vi "Save messages PGserver.vi"(7 "stop":bool, 8 "error in":errorcluster, 9 "write enable":bool=TRUE, 10 "msg":refnum<queue>, 11 "SP in":refnum<class "Save messages PGserver.lvclass">) -> (0 "error out":errorcluster, 2 "stopped":bool, 3 "SP out":refnum<class "Save messages PGserver.lvclass">)   [LabVIEW 2019, in "Save messages PGserver.lvclass"]
uses:
  Save messages PGserver.lvclass
  ctl/Save_prog_State.ctl
  Save messages PGserver.lvclass/Save messages PGserver.ctl
  PostgreSQL2LabVIEW/libpqUtility64/src/PQclose.vi
  Modbus/Eth Status/Eth Status Read Error.vi
  PostgreSQL2LabVIEW/libpqUtility64/src/PQexecute.vi
  Read conn.vi
  PostgreSQL2LabVIEW/libpqlv64/src/PQfinish.vi
  PostgreSQL2LabVIEW/libpqlv64/src/PQresultErrorMessage.vi
  PostgreSQL2LabVIEW/libpqUtility64/src/PQclear.vi
  PostgreSQL2LabVIEW/libpqlv64/src/PQsendQuery.vi
  PostgreSQL2LabVIEW/libpqlv64/src/PQgetResult.vi
  PostgreSQL2LabVIEW/libpqlv64/src/PQresultStatus.vi
  PostgreSQL2LabVIEW/libpqlv64/src/PQclear.vi
  Timer Delay/Timers.lvlib
  Modbus/Eth Status/Eth Status.lvlib
  PostgreSQL.lvlib
panel:
  out "t ms":u32
  out "State":T1=enum."requests"
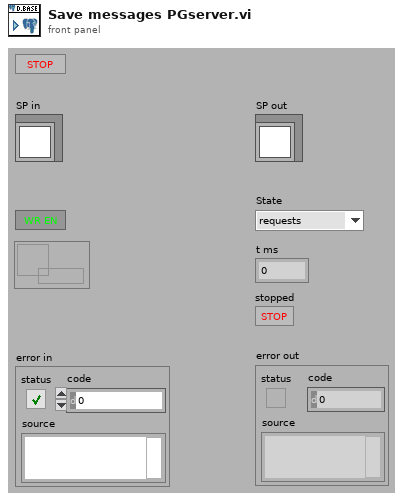
[diagram p1: front panel]
types:
  T1 = typedef "PostgreSQL.lvlib/Save_prog_State.ctl" = enum8{"initialization", "redefine", "standby", "connect", "wait to reconnect", "wait to reset timeout", "configure", "requests", "close connection", "stop"}
  T2 = typedef "Eth Status.lvlib/ICPCON Status.ctl" = cluster{"Set_state_com":refnum<data-value>, "start":refnum<data-value>, "WrEn":refnum<data-value>, "errors":refnum<data-value>, "connect":refnum<data-value>, "state":refnum<data-value>}
  T3 = typedef "PostgreSQL.lvlib/Coninfo.ctl" = cluster{"host":string, "port":string, "client_encoding":string, "dbname":string, "user":string, "password":string}
  T4 = typedef "PostgreSQL.lvlib/Save_prog_timeouts.ctl" = cluster{"reconn_timeout":i32, "read_timeout":i32, "N attempt max":i32, "t_reset_TTL":i32, "period":i32}
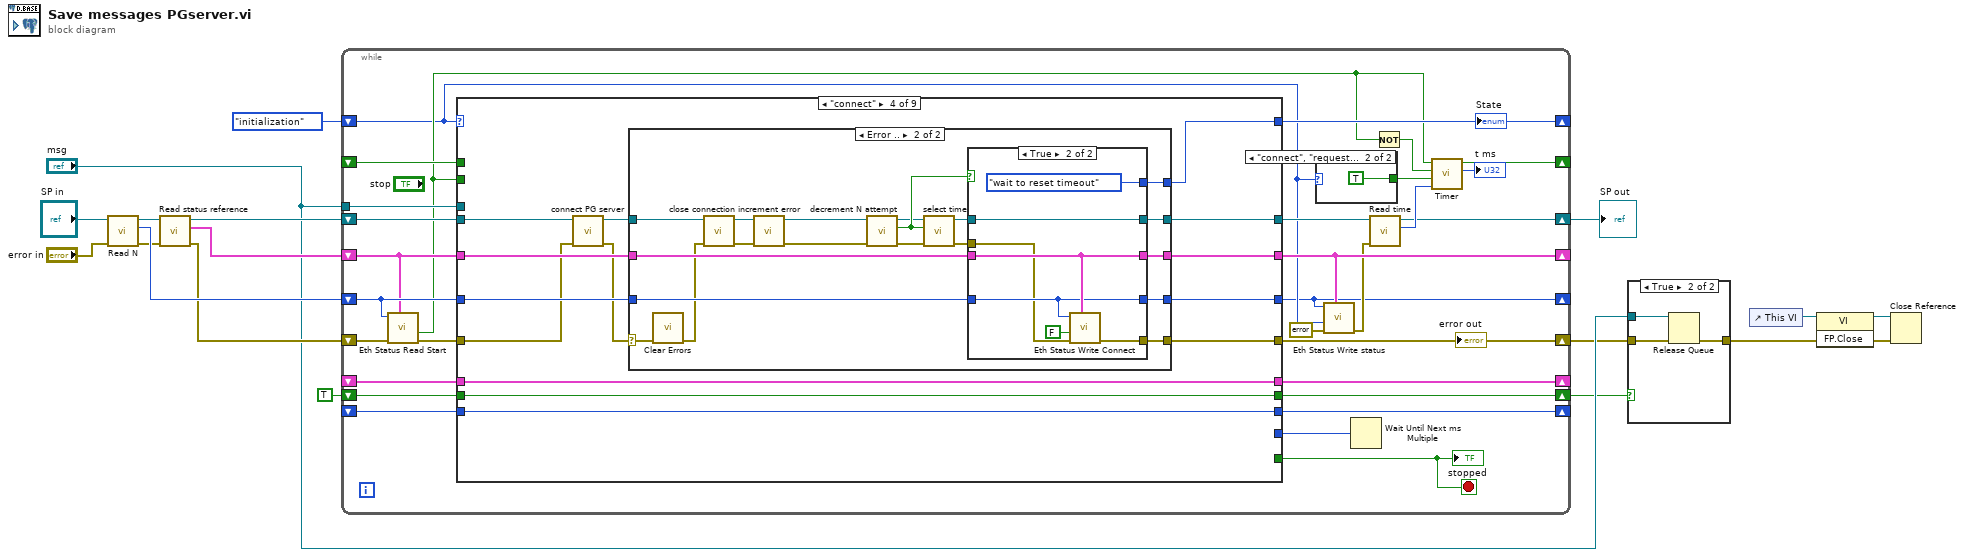
[diagram p0: block diagram]
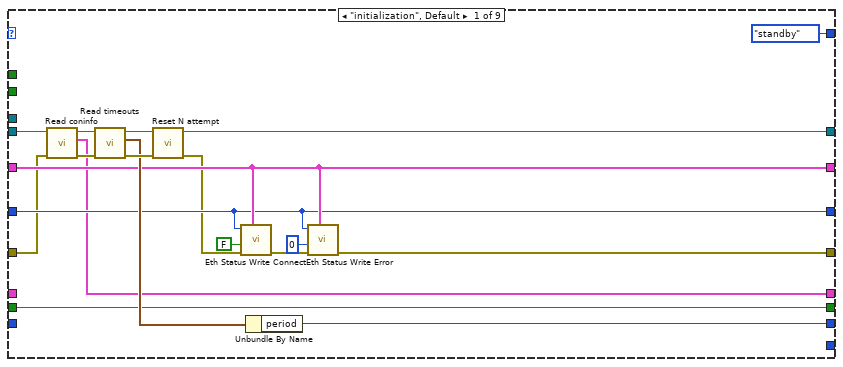
[diagram p2: hidden frame]
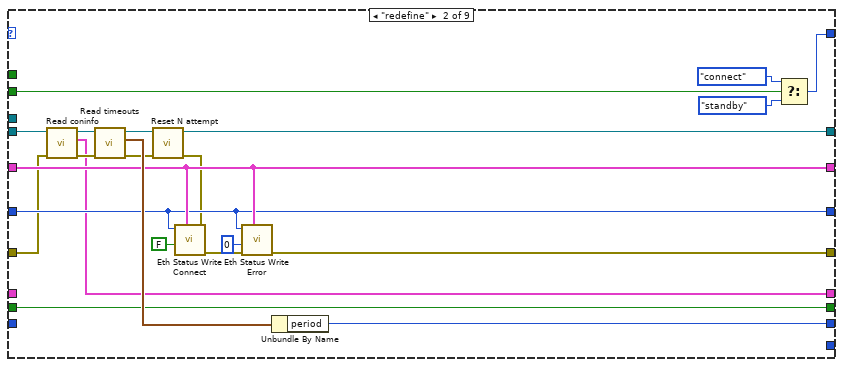
[diagram p3: hidden frame]
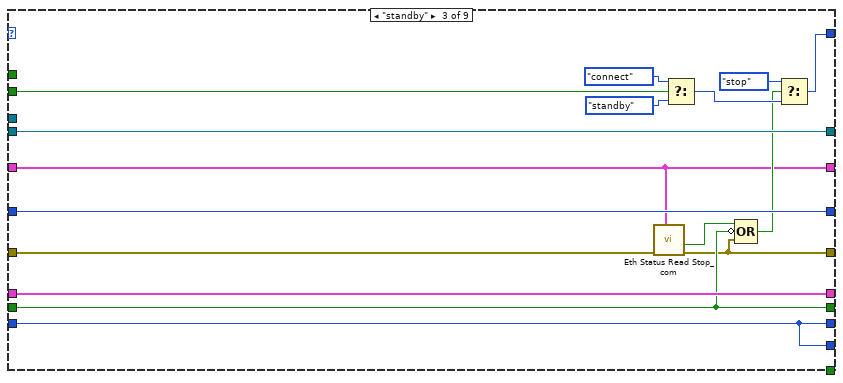
[diagram p4: hidden frame]
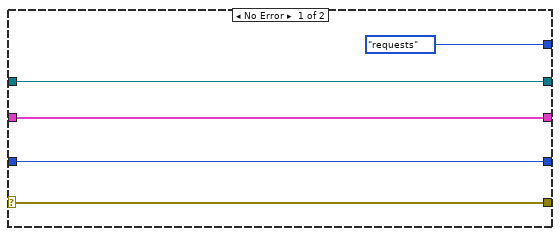
[diagram p5: hidden frame]
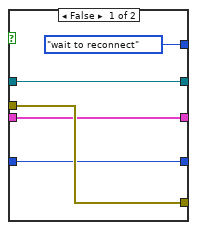
[diagram p6: hidden frame]
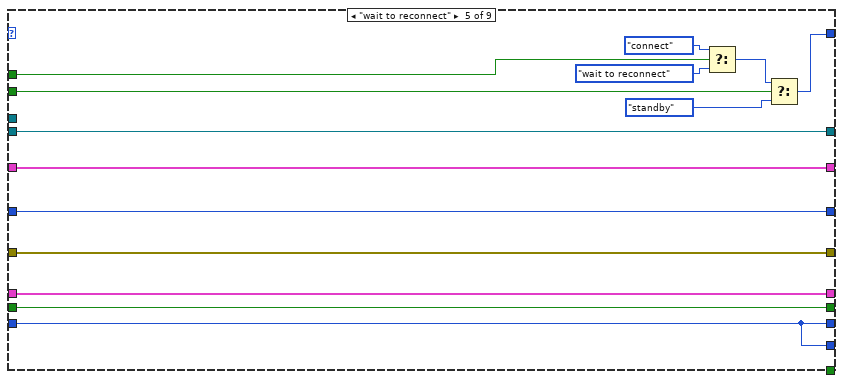
[diagram p7: hidden frame]
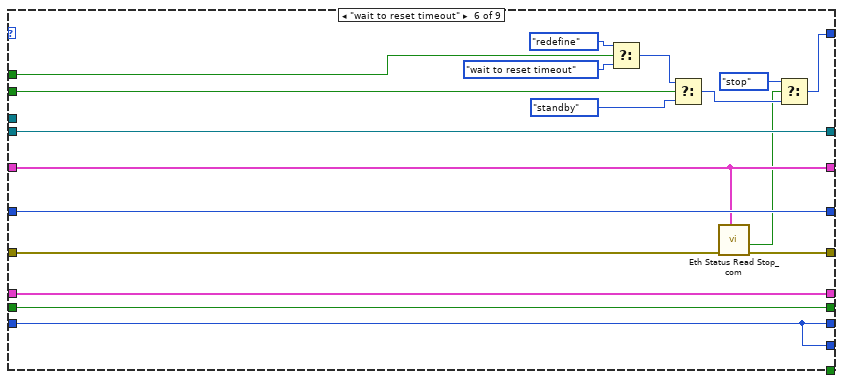
[diagram p8: hidden frame]
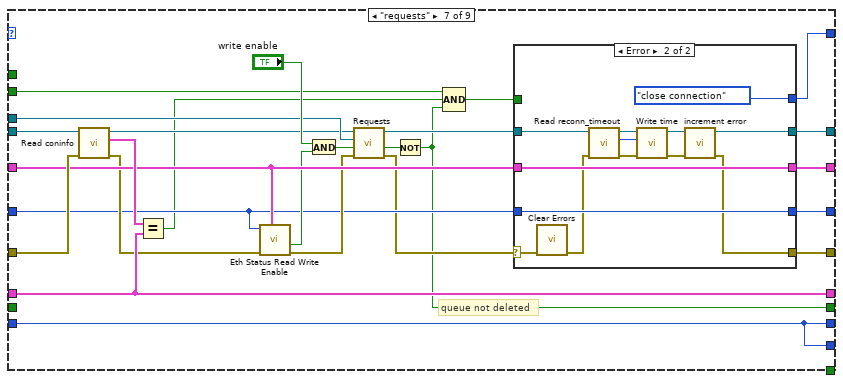
[diagram p9: hidden frame]
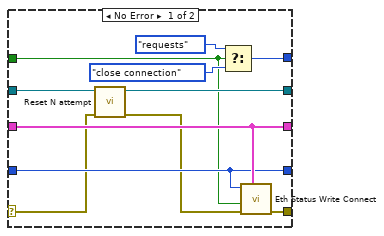
[diagram p10: hidden frame]
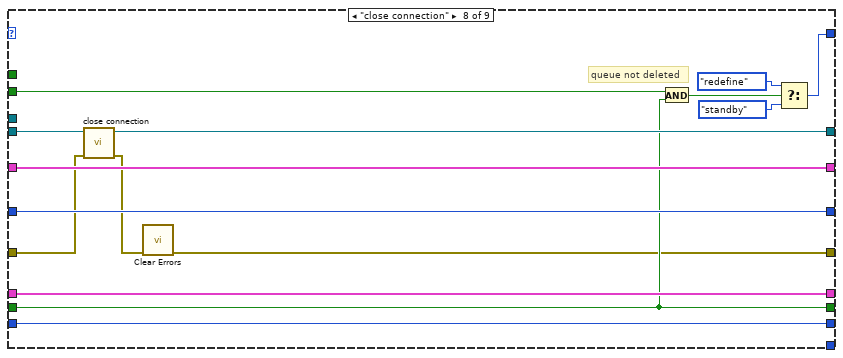
[diagram p11: hidden frame]
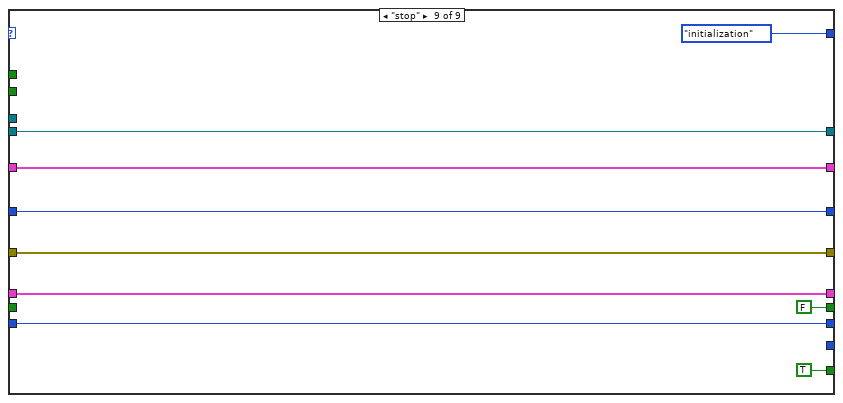
[diagram p12: hidden frame]
diagram:
  n1 = call "Read N.vi"("error in (no error)"="error in", "SP in"="SP in") -> ("error out"=w8:errorcluster, "N"=w15:i32, "SP out"=w11:refnum<class "Save messages PGserver.lvclass">)  [unwired: 7 in]
  n2 = call "Read status reference.vi"("error in (no error)"=w8, "SP in"=w11) -> ("error out"=w9:errorcluster, "Status"=w7:T2, "SP out"=w10:refnum<class "Save messages PGserver.lvclass">)  [unwired: 7 in]
  n3 = while {
    shift-right: [w45] -> _
    shift-left: _ -> [w44]
    shift-right: [w43] -> _
    shift-left: _ -> [w42]
    shift-right: [w31] -> w12
    shift-left: w10 -> [w36]
    shift-right: [w40] -> _
    shift-left: Save_prog_State."initialization" ("Save_prog_State") -> [w21]
    shift-right: [w22] -> _
    shift-left: w7 -> [w33]
    shift-right: [w18] -> _
    shift-left: w15 -> [w35]
    shift-right: [w32] -> w5
    shift-left: w9 -> [w24]
    shift-right: [w26] -> _
    shift-left: _ -> [w38]
    tunnel: "msg" -> [w30]
    shift-right: [w28] -> w4
    shift-left: TRUE -> [w27]
    stop <- w29 stop-if-true
    n4 = call "Eth Status Read Start.vi"("Status Reference"=w33, "error in (no error)"=w24, "N"=w35) -> ("error out"=w37:errorcluster, "Start"=w23:bool)  [unwired: 7 in]
    n5 = case shown="\"connect\"" w21 {
      tunnel: w23 -> [_ w88 w104 _ w168 w183 w189 w249 _]
      tunnel: w44 -> [_ _ _ _ w165 w182 _ _ _]
      tunnel: [_ _ _ _ _ _ _ _ TRUE] -> w29
      tunnel: [w51 w69 w95 w106 w157 w175 w212 w244 w254] -> w43
      tunnel: w42 -> [_ _ w95 w106 w157 w175 w212 w244 w254]
      tunnel: w36 -> [w54 w73 w101 w109 w162 w180 w194 w243 w255]
      tunnel: [w57 w75 w101 w118 w162 w180 w210 w242 w255] -> w39
      tunnel: w37 -> [w53 w72 w92 w110 w158 w172 w205 w241 w258]
      tunnel: [Save_prog_State."standby" ("Save_prog_State") w85 w98 w117 w161 w176 w209 w248 Save_prog_State."initialization" ("Save_prog_State")] -> w40
      tunnel: [w59 w78 w91 w116 w160 w170 w208 w247 w260] -> w22
      tunnel: [w58 w77 w100 w112 w159 w179 w207 w246 w259] -> w18
      tunnel: w33 -> [w59 w78 w91 w115 w160 w170 w204 w247 w260]
      tunnel: w35 -> [w58 w77 w100 w113 w159 w179 w197 w246 w259]
      tunnel: [w50 w76 w90 w114 w158 w171 w206 w237 w258] -> w32
      tunnel: [w65 w83 w93 w111 w155 w173 w187 w245 w257] -> w26
      tunnel: w38 -> [_ _ w93 w111 w155 w173 w187 w245 w257]
      tunnel: w30 -> [_ _ _ _ _ _ w196 _ _]
      tunnel: [w49 w68 w94 w105 w156 w174 w190 w239 FALSE] -> w28
      tunnel: w27 -> [w49 w68 w94 w105 w156 w174 _ w239 _]
      tunnel: [_ _ w93 _ w155 w173 w187 _ _] -> w25
      frame "initialization", Default {
        n6 = call "Read coninfo.vi"("error in (no error)"=w53, "SP in"=w54) -> ("error out"=w52:errorcluster, "conninfo"=w51:T3, "SP out"=w55:refnum<class "Save messages PGserver.lvclass">)  [unwired: 7 in]
        n7 = call "Read timeouts.vi"("error in (no error)"=w52, "SP in"=w55) -> ("error out"=w64:errorcluster, "SP timeouts"=w60:T4, "SP out"=w61:refnum<class "Save messages PGserver.lvclass">)  [unwired: 7 in]
        n8 = call "Reset N attempt.vi"("error in (no error)"=w64, "SP in"=w61) -> ("error out"=w56:errorcluster, "SP out"=w57:refnum<class "Save messages PGserver.lvclass">)  [unwired: 7 in, 1 out]
        n9 = call "Eth Status Write Connect.vi"("Status Reference"=w59, "error in (no error)"=w56, "Connect"=FALSE ("connect"), "N"=w58) -> ("error out"=w62:errorcluster)  [unwired: 7 in]
        n10 = Unbundle By Name(w60) -> ("period"=w65:i32)
        n11 = call "Eth Status Write Error.vi"("Status Reference"=w59, "error in (no error)"=w62, "Errors"=0 ("N attempt max"), "N"=w58) -> ("error out"=w50:errorcluster)  [unwired: 7 in]
      }
      frame "redefine" {
        n12 = call "Read coninfo.vi"("error in (no error)"=w72, "SP in"=w73) -> ("error out"=w71:errorcluster, "conninfo"=w69:T3, "SP out"=w70:refnum<class "Save messages PGserver.lvclass">)  [unwired: 7 in]
        n13 = call "Read timeouts.vi"("error in (no error)"=w71, "SP in"=w70) -> ("error out"=w82:errorcluster, "SP timeouts"=w84:T4, "SP out"=w81:refnum<class "Save messages PGserver.lvclass">)  [unwired: 7 in]
        n14 = call "Reset N attempt.vi"("error in (no error)"=w82, "SP in"=w81) -> ("error out"=w74:errorcluster, "SP out"=w75:refnum<class "Save messages PGserver.lvclass">)  [unwired: 7 in, 1 out]
        n15 = call "Eth Status Write Connect.vi"("Status Reference"=w78, "error in (no error)"=w74, "Connect"=FALSE ("connect"), "N"=w77) -> ("error out"=w79:errorcluster)  [unwired: 7 in]
        n16 = call "Eth Status Write Error.vi"("Status Reference"=w78, "error in (no error)"=w79, "Errors"=0 ("N attempt max"), "N"=w77) -> ("error out"=w76:errorcluster)  [unwired: 7 in]
        n17 = Unbundle By Name(w84) -> ("period"=w83:i32)
        n18 = Select(t=Save_prog_State."connect" ("Save_prog_State"), s=w88, f=Save_prog_State."standby" ("Save_prog_State")) -> (s? t:f=w85:T1)
      }
      frame "standby" {
        n19 = call "Eth Status Read Stop_com.vi"("Status Reference"=w91, "error in (no error)"=w92) -> ("error out"=w90:errorcluster, "Stop"=w89:bool)  [unwired: 8 in]
        n20 = Select(t=Save_prog_State."connect" ("Save_prog_State"), s=w104, f=Save_prog_State."standby" ("Save_prog_State")) -> (s? t:f=w97:T1)
        n21 = Compound Arithmetic op=OR(w89, invert w94, w90) -> (w96:bool)
        n22 = Select(t=Save_prog_State."stop" ("Save_prog_State"), s=w96, f=w97) -> (s? t:f=w98:T1)
      }
      frame "connect" {
        n23 = call-dynamic "connect PG server.vi"("error in (no error)"=w110, "SP in"=w109) -> ("error out"=w107:errorcluster, "SP out"=w108:refnum<class "Save messages PGserver.lvclass">)  [unwired: 7 in, 1 out]
        n24 = case shown="Error .." w107 {
          selector: w107 -> [w121 w126]
          tunnel: w108 -> [w122 w128]
          tunnel: [Save_prog_State."requests" ("Save_prog_State") w139] -> w117
          tunnel: [w122 w132] -> w118
          tunnel: [w121 w131] -> w114
          tunnel: w115 -> [w120 w133]
          tunnel: w113 -> [w119 w134]
          tunnel: [w120 w136] -> w116
          tunnel: [w119 w135] -> w112
          frame No Error {
          }
          frame Error {
            n25 = call <vilib>:"Clear Errors.vi"("error in (no error)"=w126) -> ("error out"=w125:errorcluster)  [unwired: 5 in, 1 out]
            n26 = call "close connection.vi"("error in (no error)"=w125, "SP in"=w128) -> ("error out"=w129:errorcluster, "SP out"=w130:refnum<class "Save messages PGserver.lvclass">)  [unwired: 8 in]
            n27 = call "increment error.vi"("error in (no error)"=w129, "SP in"=w130) -> ("error out"=w124:errorcluster, "SP out"=w142:refnum<class "Save messages PGserver.lvclass">)  [unwired: 7 in, 1 out]
            n28 = call "decrement N attempt.vi"("error in (no error)"=w124, "SP in"=w142) -> ("error out"=w141:errorcluster, "=0"=w140:bool, "SP out"=w127:refnum<class "Save messages PGserver.lvclass">)  [unwired: 7 in]
            n29 = call "select time.vi"("error in (no error)"=w141, "N attemt=0"=w140, "SP in"=w127) -> ("error out"=w137:errorcluster, "SP out"=w138:refnum<class "Save messages PGserver.lvclass">)  [unwired: 7 in]
            n30 = case shown="True" w140 {
              tunnel: [Save_prog_State."wait to reconnect" ("Save_prog_State") Save_prog_State."wait to reset timeout" ("Save_prog_State")] -> w139
              tunnel: w138 -> [w146 w150]
              tunnel: [w146 w150] -> w132
              tunnel: w137 -> [w145 w149]
              tunnel: [w145 w153] -> w131
              tunnel: w133 -> [w144 w152]
              tunnel: w134 -> [w143 w151]
              tunnel: [w144 w152] -> w136
              tunnel: [w143 w151] -> w135
              frame False {
              }
              frame True {
                n31 = call "Eth Status Write Connect.vi"("Status Reference"=w152, "error in (no error)"=w149, "Connect"=FALSE ("f"), "N"=w151) -> ("error out"=w153:errorcluster)  [unwired: 7 in]
              }
            }
          }
        }
      }
      frame "wait to reconnect" {
        n32 = Select(t=Save_prog_State."connect" ("Save_prog_State"), s=w165, f=Save_prog_State."wait to reconnect" ("Save_prog_State")) -> (s? t:f=w164:T1)
        n33 = Select(t=w164, s=w168, f=Save_prog_State."standby" ("Save_prog_State")) -> (s? t:f=w161:T1)
      }
      frame "wait to reset timeout" {
        n34 = Select(t=Save_prog_State."redefine" ("Save_prog_State"), s=w182, f=Save_prog_State."wait to reset timeout" ("Save_prog_State")) -> (s? t:f=w184:T1)
        n35 = Select(t=w184, s=w183, f=Save_prog_State."standby" ("Save_prog_State")) -> (s? t:f=w177:T1)
        n36 = call "Eth Status Read Stop_com.vi"("Status Reference"=w170, "error in (no error)"=w172) -> ("error out"=w171:errorcluster, "Stop"=w169:bool)  [unwired: 8 in]
        n37 = Select(t=Save_prog_State."stop" ("Save_prog_State"), s=w169, f=w177) -> (s? t:f=w176:T1)
      }
      frame "requests" {
        # "queue not deleted"
        n38 = call "Read coninfo.vi"("error in (no error)"=w205, "SP in"=w194) -> ("error out"=w203:errorcluster, "conninfo"=w211:T3, "SP out"=w193:refnum<class "Save messages PGserver.lvclass">)  [unwired: 7 in]
        n39 = Equal?(x=w211, y=w212) -> (x = y?=w188:bool)
        n40 = call "Eth Status Read Write Enable.vi"("Status Reference"=w204, "error in (no error)"=w203, "N"=w197) -> ("error out"=w201:errorcluster, "Write Enable"=w200:bool)  [unwired: 7 in]
        n41 = And(x="write enable", y=w200) -> (x .and. y?=w198:bool)
        n42 = call "Requests.vi"("error in (no error)"=w201, "write enable"=w198, "msg"=w196, "SP in"=w193) -> ("error out"=w195:errorcluster, "queue deleted"=w191:bool, "SP out"=w202:refnum<class "Save messages PGserver.lvclass">)  [unwired: 5 in]
        n43 = Not(x=w191) -> (.not. x?=w190:bool)
        n44 = Compound Arithmetic op=AND(w189, w188, w190) -> (w192:bool)
        n45 = case shown="Error" w195 {
          selector: w195 -> [w217 w226]
          tunnel: [w223 Save_prog_State."close connection" ("Save_prog_State")] -> w209
          tunnel: w192 -> [w213 _]
          tunnel: [w216 w224] -> w206
          tunnel: w204 -> [w219 w233]
          tunnel: w202 -> [w220 w228]
          tunnel: [w214 w229] -> w210
          tunnel: [w219 w233] -> w208
          tunnel: w197 -> [w218 w232]
          tunnel: [w218 w232] -> w207
          frame No Error {
            n46 = call "Reset N attempt.vi"("error in (no error)"=w217, "SP in"=w220) -> ("error out"=w215:errorcluster, "SP out"=w214:refnum<class "Save messages PGserver.lvclass">)  [unwired: 7 in, 1 out]
            n47 = Select(t=Save_prog_State."requests" ("Save_prog_State"), s=w213, f=Save_prog_State."close connection" ("Save_prog_State")) -> (s? t:f=w223:T1)
            n48 = call "Eth Status Write Connect.vi"("Status Reference"=w219, "error in (no error)"=w215, "Connect"=w213, "N"=w218) -> ("error out"=w216:errorcluster)  [unwired: 7 in]
          }
          frame Error {
            n49 = call <vilib>:"Clear Errors.vi"("error in (no error)"=w226) -> ("error out"=w225:errorcluster)  [unwired: 5 in, 1 out]
            n50 = call "Read reconn_timeout.vi"("error in (no error)"=w225, "SP in"=w228) -> ("error out"=w234:errorcluster, "reconn_timeout"=w235:i32, "SP out"=w227:refnum<class "Save messages PGserver.lvclass">)  [unwired: 7 in]
            n51 = call "Write time.vi"("error in (no error)"=w234, "time"=w235, "SP in"=w227) -> ("error out"=w230:errorcluster, "SP out"=w231:refnum<class "Save messages PGserver.lvclass">)  [unwired: 7 in]
            n52 = call "increment error.vi"("error in (no error)"=w230, "SP in"=w231) -> ("error out"=w224:errorcluster, "SP out"=w229:refnum<class "Save messages PGserver.lvclass">)  [unwired: 7 in, 1 out]
          }
        }
      }
      frame "close connection" {
        # "queue not deleted"
        n53 = call "close connection.vi"("error in (no error)"=w241, "SP in"=w243) -> ("error out"=w238:errorcluster, "SP out"=w242:refnum<class "Save messages PGserver.lvclass">)  [unwired: 8 in]
        n54 = call <vilib>:"Clear Errors.vi"("error in (no error)"=w238) -> ("error out"=w237:errorcluster)  [unwired: 5 in, 1 out]
        n55 = And(x=w249, y=w239) -> (x .and. y?=w240:bool)
        n56 = Select(t=Save_prog_State."redefine" ("Save_prog_State"), s=w240, f=Save_prog_State."standby" ("Save_prog_State")) -> (s? t:f=w248:T1)
      }
      frame "stop" {
      }
    }
    "stopped" <- w29
    "error out" <- w32
    "State" <- w40
    n57 = case shown="\"connect\", \"requests\"" w21 {
      tunnel: [_ TRUE] -> w46
      frame "initialization", Default {
      }
      frame "connect", "requests" {
      }
    }
    n58 = call "Eth Status Write status.vi"("Status Reference"=w22, "error in (no error)"=errorcluster {"status"=FALSE, "code"=0, "source"=""}, "status"=w21, "N"=w18) -> ("error out"=w20:errorcluster)  [unwired: 7 in]
    n59 = Wait Until Next ms Multiple(millisecond multiple=w25) -> ()  [unwired: 1 out]
    n60 = call "Read time.vi"("error in (no error)"=w20, "SP in"=w39) -> ("time"=w41:i32, "SP out"=w31:refnum<class "Save messages PGserver.lvclass">)  [unwired: 7 in, 1 out]
    n61 = Not(x=w23) -> (.not. x?=w47:bool)
    n62 = call "Timer.vi"("ms"=w41, "Load (F)"=w46, "Reset (F)"=w47, "Start (T)"=w23) -> ("t ms"=→"t ms":u32, "End"=w45:bool)  [unwired: 5 in]
  }
  "SP out" <- w12
  n63 = case shown="True" w4 {
    tunnel: "msg" -> [_ w265]
    tunnel: w5 -> [w262 w264]
    tunnel: [w262 w263] -> w3
    frame False {
    }
    frame True {
      n64 = Release Queue(queue=w265, error in (no error)=w264) -> (error out=w263:errorcluster)  [unwired: 1 in, 2 out]
    }
  }
  n65 = control-ref of="This VI"() -> (w2:refnum<vi>)
  n66 = invoke class="VI" method="FP.Close"(reference=w2) -> (reference out=w1:refnum<vi>)  [unwired: 2 in, 2 out]
  n67 = Close Reference(reference=w1, error in (no error)=w3) -> ()  [unwired: 1 out]
